vi "Rename Exp.vi"(8 "error in (no error)":errorcluster, 10 "New exp name":string, 11 "Control-Client in":refnum<class "Control-Client.lvclass">) -> (0 "error out":errorcluster, 3 "Control-Client out":refnum<class "Control-Client.lvclass">)   [LabVIEW 2019, in "Control-Client.lvclass"]
uses:
  Control-Client.lvclass
  Experiments/Experiment.lvclass
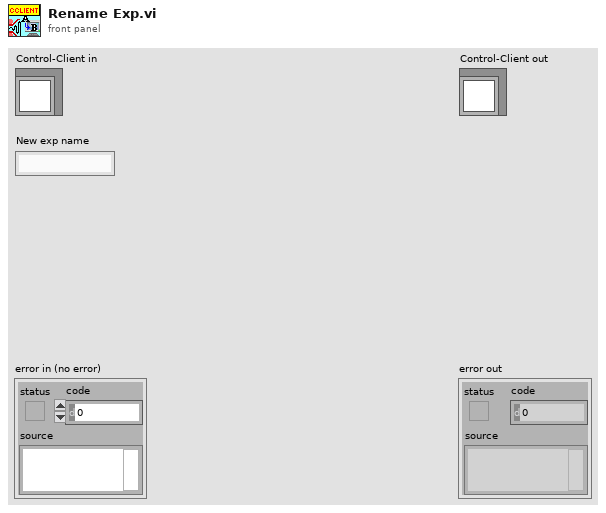
[diagram p1: front panel]
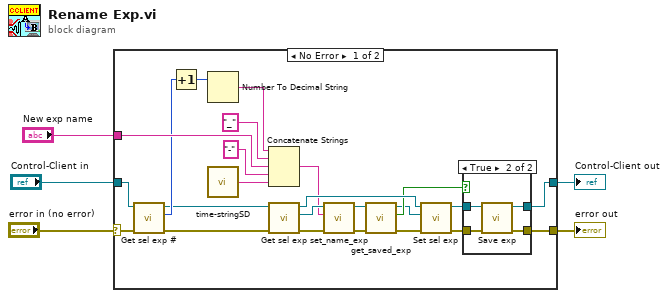
[diagram p0: block diagram]
diagram:
  n1 = case shown="No Error" "error in (no error)" {
    selector: "error in (no error)" -> [w14 w37]
    tunnel: [w10 w37] -> w4
    tunnel: [w29 w36] -> w2
    tunnel: "Control-Client in" -> [w15 w36]
    tunnel: "New exp name" -> [w17 _]
    frame No Error {
      n2 = call "Get sel exp #.vi"("error in (no error)"=w14, "Control-Client in"=w15) -> ("error out"=w11:errorcluster, "Exp sel #"=w13:i32, "Control-Client out"=w12:refnum<class "Control-Client.lvclass">)  [unwired: 7 in]
      n3 = Increment(x=w13) -> (x+1=w22:i32)
      n4 = Number To Decimal String(number=w22) -> (decimal integer string=w20:string)  [unwired: 1 in]
      n5 = call "time-stringSD.vi"() -> ("time"=w18:string)
      n6 = Concatenate Strings(w20, "_" ("string"), w17, "-" ("string"), w18) -> (w16:string)
      n7 = call "Get sel exp.vi"("error in (no error)"=w11, "Control-Client in"=w12) -> ("error out"=w28:errorcluster, "Sel experiment"=w27:refnum<class "Experiment.lvclass">, "Control-Client out"=w26:refnum<class "Control-Client.lvclass">)  [unwired: 7 in]
      n8 = call "set_name_exp.vi"("error in (no error)"=w28, "Exp name"=w16, "Experiment.lvclass in"=w27) -> ("error out"=w8:errorcluster, "Experiment.lvclass out"=w25:refnum<class "Experiment.lvclass">)  [unwired: 7 in]
      n9 = call "get_saved_exp.vi"("error in (no error)"=w8, "Experiment.lvclass in"=w25) -> ("error out"=w7:errorcluster, "Saved"=w24:bool, "Experiment.lvclass out"=w9:refnum<class "Experiment.lvclass">)  [unwired: 7 in]
      n10 = call "Set sel exp.vi"("error in (no error)"=w7, "Experiment"=w9, "Control-Client in"=w26) -> ("error out"=w6:errorcluster, "Control-Client out"=w23:refnum<class "Control-Client.lvclass">)  [unwired: 7 in]
      n11 = case shown="True" w24 {
        tunnel: [w31 w35] -> w29
        tunnel: [w30 w34] -> w10
        tunnel: w23 -> [w31 w33]
        tunnel: w6 -> [w30 w32]
        frame False {
        }
        frame True {
          n12 = call "Save exp.vi"("error in (no error)"=w32, "Control-Client in"=w33) -> ("error out"=w34:errorcluster, "Control-Client out"=w35:refnum<class "Control-Client.lvclass">)  [unwired: 8 in]
        }
      }
    }
    frame Error {
    }
  }
  "error out" <- w4
  "Control-Client out" <- w2
